vi "Create Local Events.vi"() -> (0 "error out":errorcluster, 3 "Local Events":T1)   [LabVIEW 2020, in "TDS1002 Oscilloscope.lvlib" / "Local Events.lvlib"]
doc: "____\nPantherLAB Templates 1.0.0.5\nCopyright (c) 2022, PantherLAB\n\n<b>Note:</b> This VI was modified by the <b>Validate DQMH Module</b> tool to be shared clone reentrant."
uses:
  Local Events.lvlib
  Local Events--cluster.ctl
  Helper loop arguments--cluster.ctl
  TDS1002 Oscilloscope.lvlib
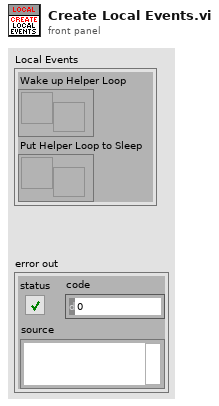
[diagram p1: front panel]
types:
  T1 = typedef "TDS1002 Oscilloscope.lvlib/Local Events.lvlib/Local Events--cluster.ctl" = cluster{"Wake up Helper Loop":refnum<user-event>, "Put Helper Loop to Sleep":refnum<user-event>}
  T2 = typedef "TDS1002 Oscilloscope.lvlib/Helper loop arguments--cluster.ctl" = cluster{"Helper Loop Timeout":i32, "VISA resource name":refnum<visa-resource-name>}
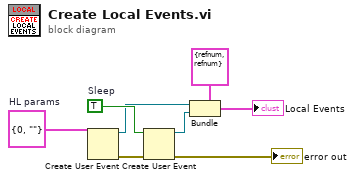
[diagram p0: block diagram]
diagram:
  w2 = T2 {"Helper Loop Timeout"=0, "VISA resource name"=""}  # HL params
  w6 = TRUE  # Sleep
  n1 = Create User Event(user event datatype=w2) -> (user event=w1:refnum<user-event>, error out=w8:errorcluster)  [unwired: 1 in]
  n2 = Create User Event(user event datatype=w6, error in=w8) -> (user event=w5:refnum<user-event>, error out=→"error out":errorcluster)
  n3 = Bundle(cluster=T1 {"Wake up Helper Loop"=refnum, "Put Helper Loop to Sleep"=refnum} ("Local Events"), "Wake up Helper Loop"=w1, "Put Helper Loop to Sleep"=w5) -> (→"Local Events":T1)
